vi "update.vi"(8 "error in (no error)":errorcluster, 11 "StaticOutputEditor in":refnum<class "StaticOutputEditor.lvclass">) -> (0 "error out":errorcluster, 3 "StaticOutputEditor out":refnum<class "StaticOutputEditor.lvclass">)   [LabVIEW 2011, in "Views.lvlib" / "ScriptEditor.lvlib" / "StaticOutputEditor.lvclass"]
uses:
  StaticOutputEditor.lvclass
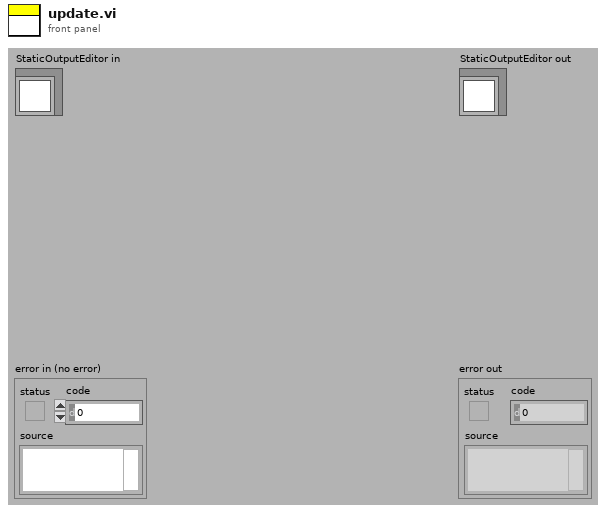
[diagram p1: front panel]
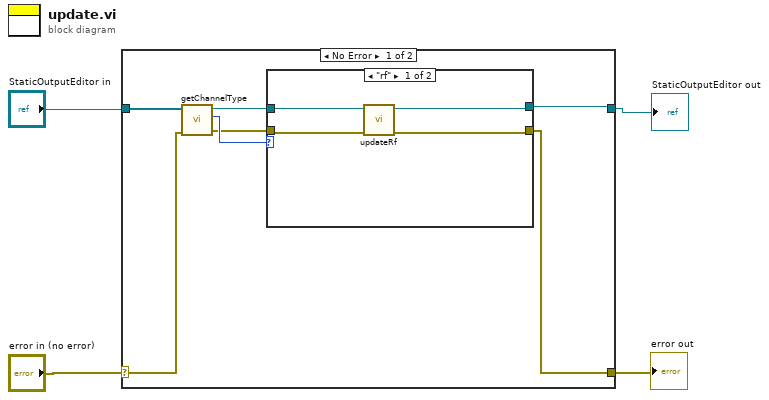
[diagram p0: block diagram]
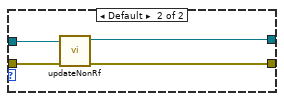
[diagram p2: hidden frame]
diagram:
  n1 = case shown="No Error" "error in (no error)" {
    selector: "error in (no error)" -> [w10 w21]
    tunnel: [w5 w21] -> w3
    tunnel: [w6 w20] -> w1
    tunnel: "StaticOutputEditor in" -> [w11 w20]
    frame No Error {
      n2 = call "getChannelType.vi"("error in (no error)"=w10, "StaticOutputEditor in"=w11) -> ("error out"=w7:errorcluster, "channel_type"=w9:enum16{"ao", "do", "ai", "di", "rf"}, "StaticOutputEditor out"=w8:refnum<class "StaticOutputEditor.lvclass">)  [unwired: 7 in]
      n3 = case shown="\"rf\"" w9 {
        tunnel: w8 -> [w15 w19]
        tunnel: w7 -> [w14 w18]
        tunnel: [w13 w17] -> w6
        tunnel: [w12 w16] -> w5
        frame "rf" {
          n4 = call "updateRf.vi"("error in (no error)"=w14, "StaticOutputEditor in"=w15) -> ("error out"=w12:errorcluster, "StaticOutputEditor out"=w13:refnum<class "StaticOutputEditor.lvclass">)  [unwired: 8 in]
        }
        frame Default {
          n5 = call "updateNonRf.vi"("error in (no error)"=w18, "StaticOutputEditor in"=w19) -> ("error out"=w16:errorcluster, "StaticOutputEditor out"=w17:refnum<class "StaticOutputEditor.lvclass">)  [unwired: 8 in]
        }
      }
    }
    frame Error {
    }
  }
  "error out" <- w3
  "StaticOutputEditor out" <- w1
